vi "Add.vi"(8 "error in (no error)":errorcluster caption="错误输入（无错误）", 9 "Value":variant, 10 "Key":variant, 11 "HashTable 输入":refnum<class "HashTable.lvclass"> caption="DNL_LabVIEW Object in") -> (0 "error out":errorcluster caption="错误输出", 3 "HashTable 输出":refnum<class "HashTable.lvclass"> caption="DNL_LabVIEW Object out")   [LabVIEW 2012, in "HashTable.lvclass"]
uses:
  HashTable.lvclass
  HashTable.lvclass/HashTable.ctl
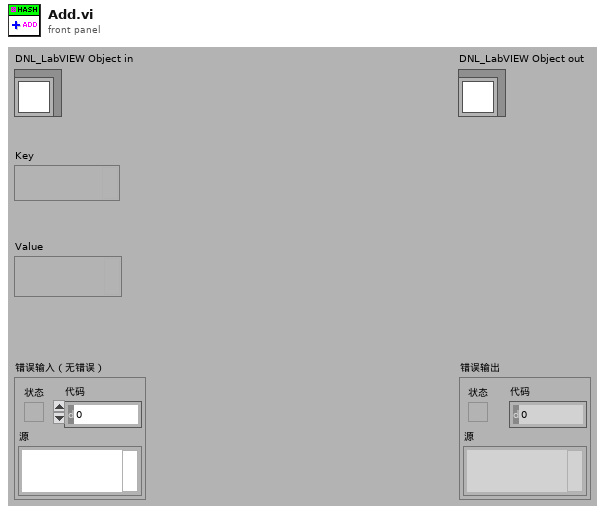
[diagram p1: front panel]
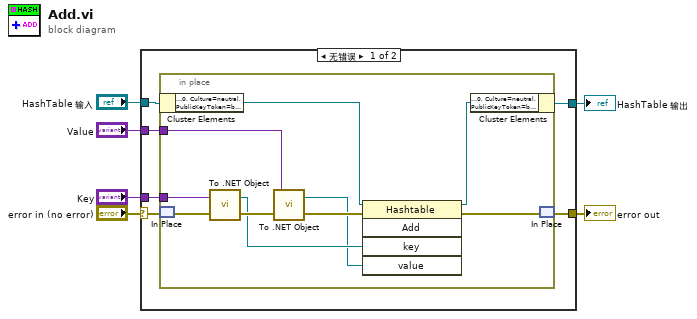
[diagram p0: block diagram]
diagram:
  n1 = case shown="无错误" "error in (no error)" {
    selector: "error in (no error)" -> [w12 w24]
    tunnel: [w11 w24] -> w5
    tunnel: [w7 w23] -> w3
    tunnel: "HashTable 输入" -> [w10 w23]
    tunnel: "Key" -> [w9 _]
    tunnel: "Value" -> [w8 _]
    frame No Error {
      n2 = in-place {
        in-place-border: w9 -> [w16]
        in-place-border: w8 -> [w14]
        n3 = in-place-cluster #1(w10) -> ("HashTable"=w22:refnum<k24>)
        n4 = in-place-match #2(w12) -> (w19:errorcluster)
        n5 = call <vilib>:"To .NET Object.vi"("error in (no error)"=w19, "anything"=w16) -> ("error out"=w18:errorcluster, ".NET object"=w15:refnum<k24>)
        n6 = call <vilib>:"To .NET Object.vi"("error in (no error)"=w18, "anything"=w14) -> ("error out"=w17:errorcluster, ".NET object"=w13:refnum<k24>)
        n7 = invoke class="Hashtable" method="Add"(reference=w22, error in=w17, "key"=w15, "value"=w13) -> (reference out=w21:refnum<k24>, error out=w20:errorcluster)  [unwired: 1 in, 3 out]
        n8 = in-place-cluster #1("HashTable"=w21) -> (w7:refnum<class "HashTable.lvclass">)
        n9 = in-place-match #2(w20) -> (w11:errorcluster)
      }
    }
    frame Error {
    }
  }
  "error out" <- w5
  "HashTable 输出" <- w3
